vi "Main.vi"() -> ()   [LabVIEW 2018, in "Bookmark Manager.lvlib"]
uses:
  Bookmark Manager.lvlib
  Controls/State.ctl
  Controls/Bookmarks Groups.ctl
  Controls/Application Information.ctl
  Controls/VI Information.ctl
  Controls/VI Bookmark.ctl
  <vilib>/event_ctls.llb/eventvkey.ctl
panel:
  in  "Bookmarks Group":T1
  in  "Help":bool
  in  "Close":bool
  in  "Bookmarks":string(tree)
  in  "Scope":u16(ring) items=["Main Application Instance", "Eulogy", "Default Bookmark Manager with image"]
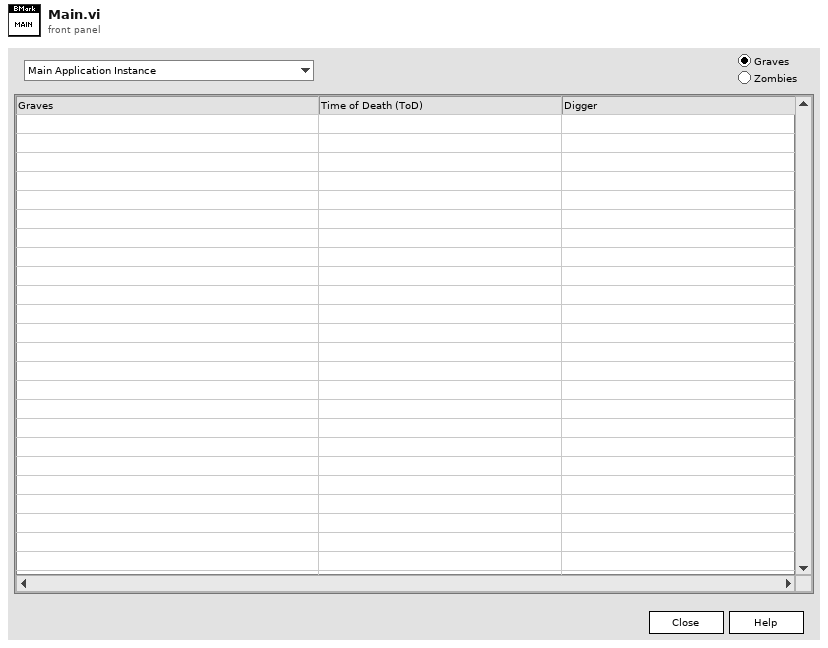
[diagram p1: front panel]
types:
  T1 = typedef "Bookmark Manager.lvlib/Bookmarks Groups.ctl" = enum32{"Graves", "Zombies"}
  T2 = typedef "Bookmark Manager.lvlib/State.ctl" = cluster{"Bookmarks":T3[], "Bookmarks Filter":T1, "Bookmarks Group":refnum<vi>, "Bookmarks View":refnum<vi>, "Front Panel":refnum<vi>, "Scopes":refnum<vi>}
  T3 = typedef "Bookmark Manager.lvlib/VI Bookmark.ctl" = cluster{"Bookmark Info":cluster{"Bookmark ID":u32, "Bookmark Tag":string, "Label Text":string}, "VI Info":T4}
  T4 = typedef "Bookmark Manager.lvlib/VI Information.ctl" = cluster{"App Info":T5, "Name":string, "Path":path}
  T5 = typedef "Bookmark Manager.lvlib/Application Information.ctl" = cluster{"Project":string, "Target":string}
  T6 = enum32{"Invalid", "Standard", "Closed", "Hidden", "Minimized", "Maximized"}
  T7 = typedef "eventvkey.ctl" = enum16{"ASCII", "Enter", "Return", "Shift", "Ctrl", "Alt", "Cmd", "Opt", "Caps", "NumLock", "Clear", "Break", "Up", "Down", "Left", "Right", "Insert", "Delete", "Home", "End", "PageUp", "PageDown", "Escape", "Help", "Pause", "ScrollLock", "F1", "F2", "F3", "F4", "F5", "F6", "F7", "F8", "F9", "F10", "F11", "F12", "F13", "F14", "F15", "F16", "F17", "F18", "F19", "F20", "F21", "F22", "F23", "F24", "Play", "VolumeUp", "VolumeDown", "Mute", "Two Byte Char"}
  T8 = typedef "LVPoint32TypeDef.ctl" = cluster{"Horizontal":i32, "Vertical":i32}
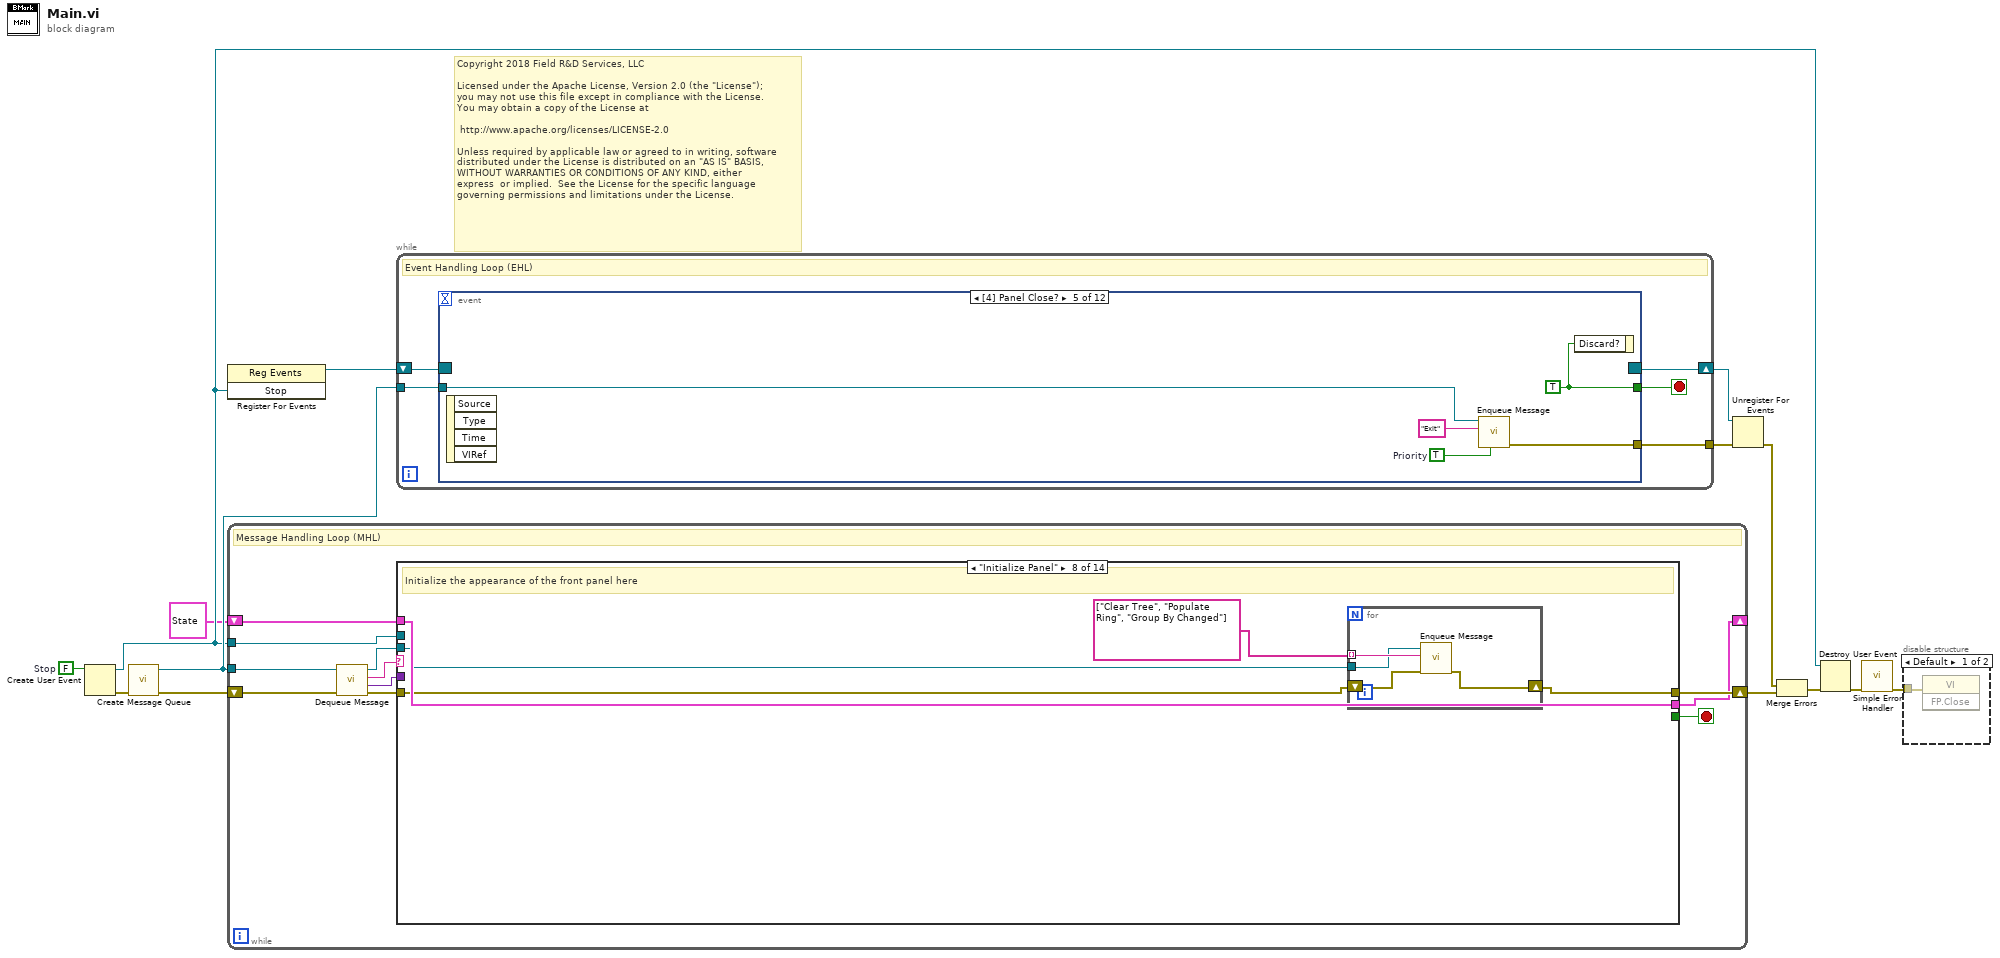
[diagram p0: block diagram]
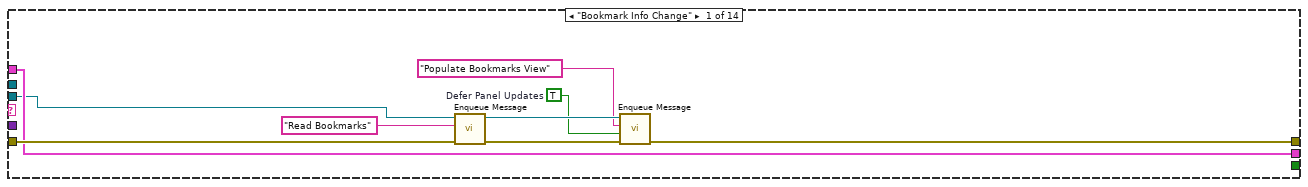
[diagram p3: hidden frame]
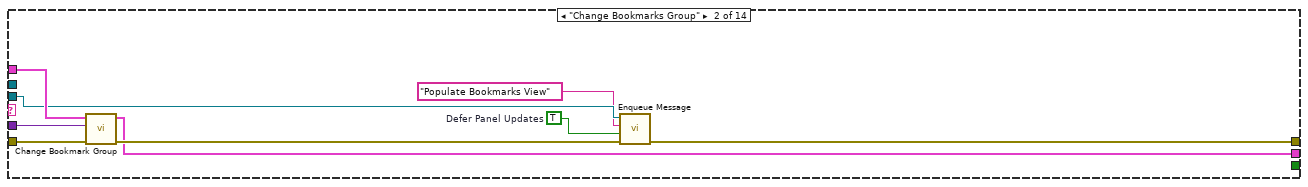
[diagram p4: hidden frame]
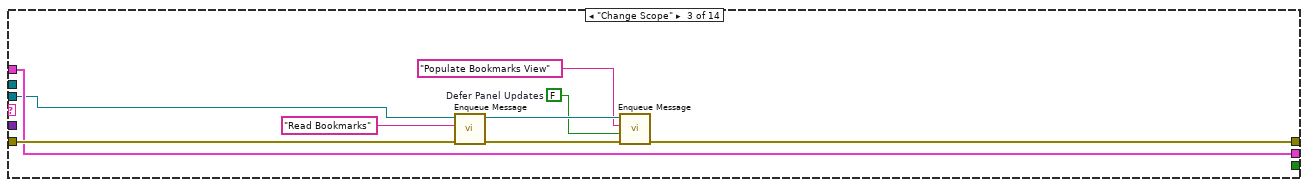
[diagram p5: hidden frame]
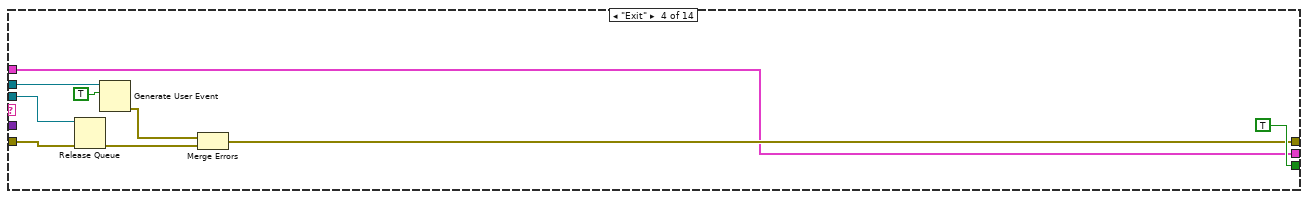
[diagram p6: hidden frame]
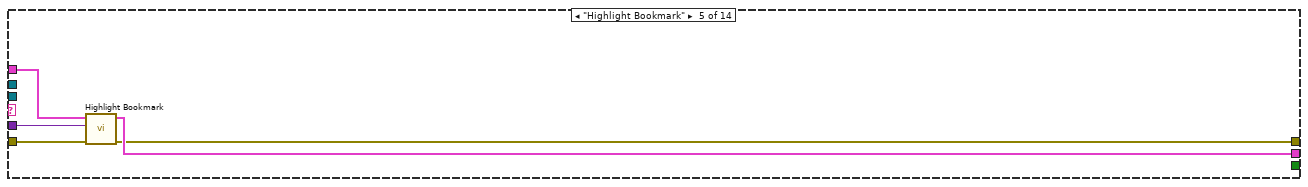
[diagram p7: hidden frame]
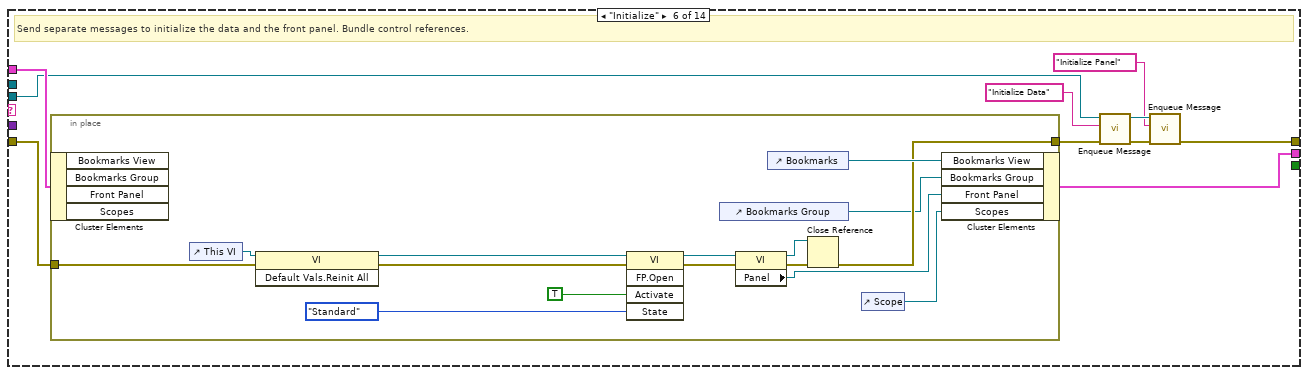
[diagram p8: hidden frame]
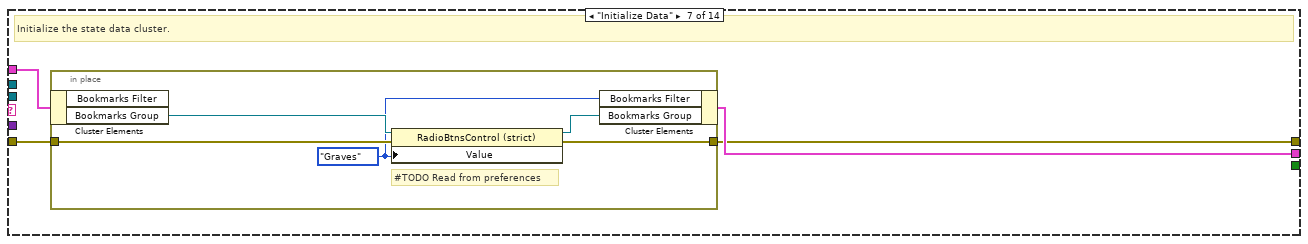
[diagram p9: hidden frame]
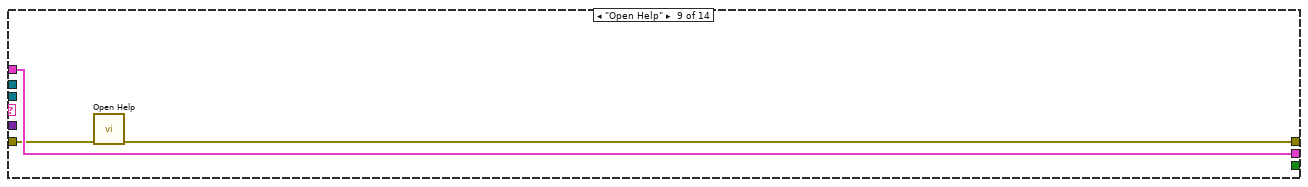
[diagram p10: hidden frame]
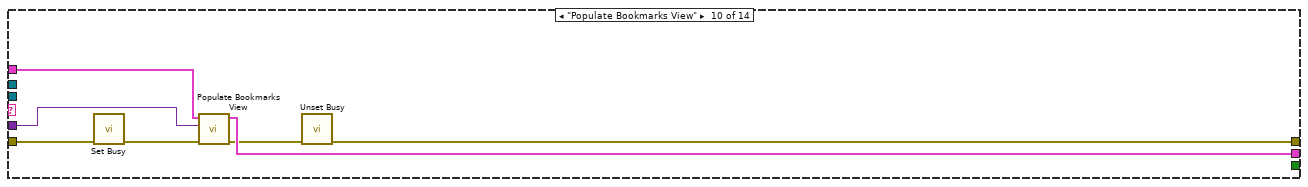
[diagram p11: hidden frame]
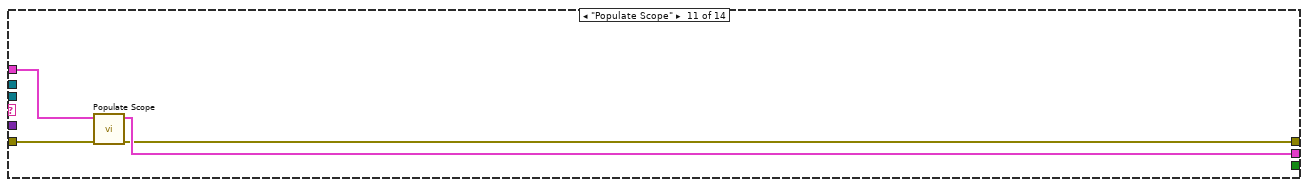
[diagram p12: hidden frame]
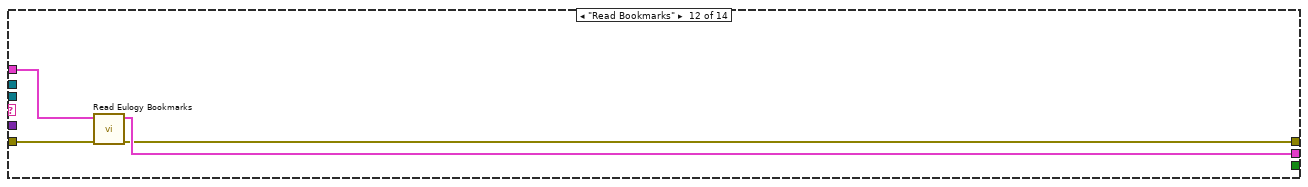
[diagram p13: hidden frame]
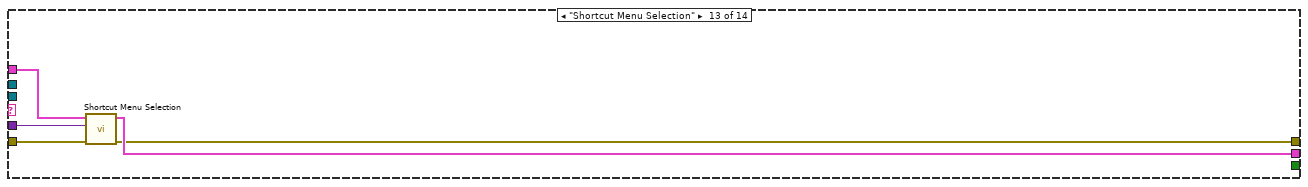
[diagram p14: hidden frame]
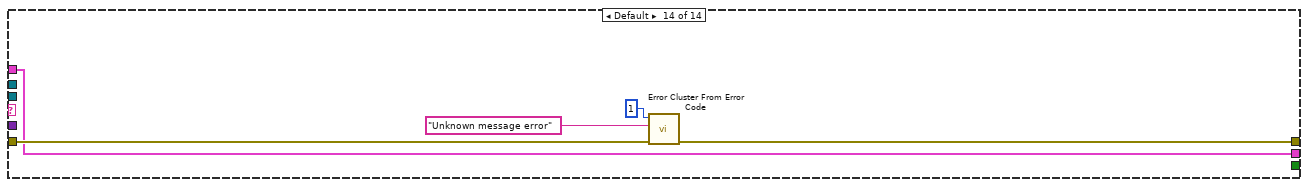
[diagram p15: hidden frame]
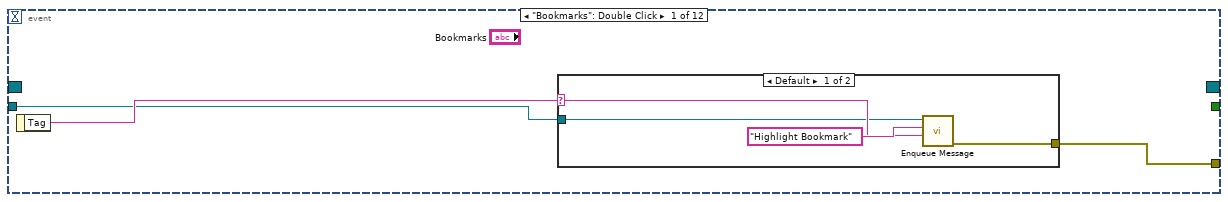
[diagram p16: hidden frame]
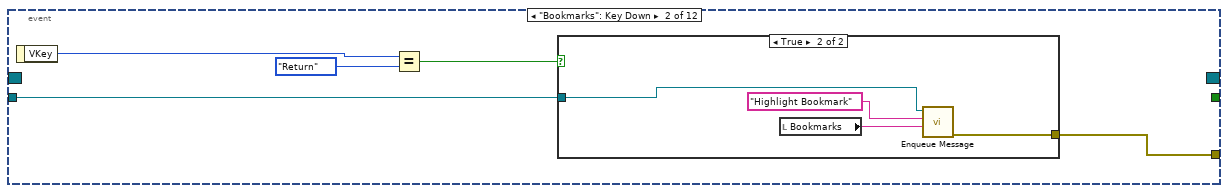
[diagram p18: hidden frame]
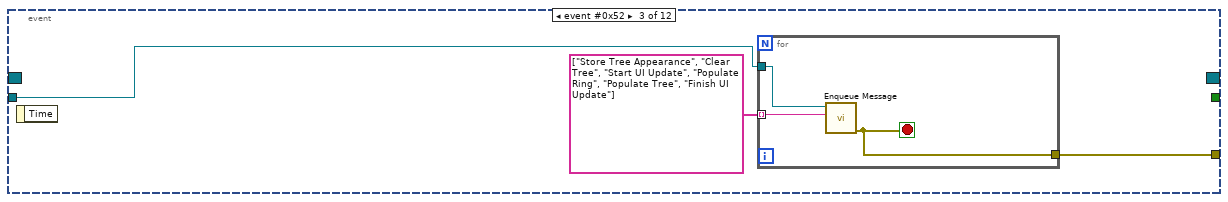
[diagram p20: hidden frame]
diagram:
  w12 = FALSE  # Stop
  # "Copyright 2018 Field R&D Services, LLC\n\nLicensed under the Apache License, Version 2.0 (the \"License\");\nyou may not use this file except in compliance with the License.\nYou may obtain a copy of the License at\n\n\thttp://www.apache.org/licenses/LICENSE-2.0\n\nUnless required by applicable law or agreed to in writing, software\ndistributed under the License is distributed on an \"AS IS\" BASIS,\nWITHOUT WARRANTIES OR CONDITIONS OF ANY KIND, either \nexpress  or implied.  See the License for the specific language \ngoverning permissions and limitations under the License."
  n1 = Create User Event(user event datatype=w12) -> (user event=w5:refnum<user-event>, error out=w11:errorcluster)  [unwired: 1 in]
  n2 = call "Create Message Queue.vi"("Error In"=w11) -> ("Error Out"=w9:errorcluster, "Message Queue"=w10:refnum<queue>)  [unwired: 9 in]
  n3 = register-events(w5) -> (reference out=w14:refnum<event-registration>)  [unwired: 2 in, 1 out]
  n4 = while {
    tunnel: w10 -> [w25]
    shift-right: [w23] -> w7
    shift-left: w9 -> [w22]
    tunnel: w5 -> [w19]
    shift-right: [w16] -> _
    shift-left: T2 {"Bookmarks"=[], "Bookmarks Filter"=enum."Graves", "Bookmarks Group"=refnum, "Bookmarks View"=refnum, "Front Panel"=refnum, "Scopes"=refnum} ("State") -> [w17]
    stop <- w20 stop-if-true
    # "Message Handling Loop (MHL)"
    n5 = call "Dequeue Message.vi"("Error In"=w22, "Message Queue In"=w25) -> ("Error Out"=w21:errorcluster, "Data"=w15:variant, "Command"=w24:string, "Message Queue Out"=w18:refnum<queue>)  [unwired: 6 in]
    n6 = case shown="\"Initialize Panel\"" w24 {
      tunnel: [w28 w38 w47 w59 w63 w68 w92 w101 w110 w114 w120 w124 w129 w133] -> w23
      tunnel: w21 -> [w34 w43 w52 w61 w66 w73 w93 w102 w111 w117 w121 w125 w132 w135]
      tunnel: [_ _ _ TRUE _ _ _ _ _ _ _ _ _ _] -> w20
      tunnel: w19 -> [_ _ _ w58 _ _ _ _ _ _ _ _ _ _]
      tunnel: w18 -> [w32 w37 w50 w54 _ w74 _ w103 _ _ _ _ _ _]
      tunnel: w17 -> [w33 w40 w51 w53 w62 w76 w95 w105 w112 w119 w123 w127 w131 w134]
      tunnel: [w33 w39 w51 w53 w64 w75 w94 w105 w112 w118 w122 w126 w130 w134] -> w16
      tunnel: w15 -> [_ w41 _ _ w65 _ _ _ _ w113 _ _ w128 _]
      frame "Bookmark Info Change" {
        w26 = TRUE  # Defer Panel Updates
        n7 = call "Enqueue Message.vi"("Error In"=w34, "Command"="Read Bookmarks", "Message Queue In"=w32) -> ("Error Out"=w30:errorcluster, "Message Queue Out"=w29:refnum<queue>)  [unwired: 7 in]
        n8 = call "Enqueue Message.vi"("Error In"=w30, "Data"=w26, "Command"="Populate Bookmarks View", "Message Queue In"=w29) -> ("Error Out"=w28:errorcluster)  [unwired: 6 in, 1 out]
      }
      frame "Change Bookmarks Group" {
        w35 = TRUE  # Defer Panel Updates
        n9 = call "Change Bookmark Group.vi"("Error In"=w43, "Data"=w41, "State In"=w40) -> ("Error Out"=w42:errorcluster, "State Out"=w39:T2)  [unwired: 7 in]
        n10 = call "Enqueue Message.vi"("Error In"=w42, "Data"=w35, "Command"="Populate Bookmarks View", "Message Queue In"=w37) -> ("Error Out"=w38:errorcluster)  [unwired: 6 in, 1 out]
      }
      frame "Change Scope" {
        w44 = FALSE  # Defer Panel Updates
        n11 = call "Enqueue Message.vi"("Error In"=w52, "Command"="Read Bookmarks", "Message Queue In"=w50) -> ("Error Out"=w48:errorcluster, "Message Queue Out"=w49:refnum<queue>)  [unwired: 7 in]
        n12 = call "Enqueue Message.vi"("Error In"=w48, "Data"=w44, "Command"="Populate Bookmarks View", "Message Queue In"=w49) -> ("Error Out"=w47:errorcluster)  [unwired: 6 in, 1 out]
      }
      frame "Exit" {
        n13 = Release Queue(queue=w54, error in (no error)=w61) -> (error out=w55:errorcluster)  [unwired: 1 in, 2 out]
        n14 = Generate User Event(user event=w58, event data cluster=TRUE ("event data")) -> (error out=w56:errorcluster)  [unwired: 2 in, 1 out]
        n15 = Merge Errors(w56, w55) -> (w59:errorcluster)
      }
      frame "Highlight Bookmark" {
        n16 = call "Highlight Bookmark.vi"("Error In"=w66, "Data"=w65, "State In"=w62) -> ("Error Out"=w63:errorcluster, "State Out"=w64:T2)  [unwired: 7 in]
      }
      frame "Initialize" {
        # "Send separate messages to initialize the data and the front panel. Bundle control references."
        n17 = in-place {
          in-place-border: w73 -> [w88]
          in-place-border: [w84] -> w72
          n18 = in-place-cluster #1(w76) -> ()  [unwired: 4 out]
          n19 = control-ref of="This VI"() -> (w85:refnum<vi>)
          n20 = invoke class="VI" method="Default Vals.Reinit All"(reference=w85, error in=w88) -> (reference out=w87:refnum<vi>, error out=w78:errorcluster)  [unwired: 1 in, 1 out]
          n21 = invoke class="VI" method="FP.Open"(reference=w87, error in=w78, "Activate"=TRUE ("Activate?"), "State"=T6."Standard") -> (reference out=w82:refnum<vi>, error out=w81:errorcluster)  [unwired: 1 in, 3 out]
          n22 = control-ref of="Bookmarks Group"() -> (w77:refnum<vi>)
          n23 = property class="VI"(reference=w82, error in=w81) -> (reference out=w83:refnum<vi>, error out=w86:errorcluster, "Panel"=w89:refnum<vi>)
          n24 = control-ref of="Bookmarks"() -> (w91:refnum<vi>)
          n25 = Close Reference(reference=w83, error in (no error)=w86) -> (error out=w84:errorcluster)
          n26 = control-ref of="Scope"() -> (w90:refnum<vi>)
          n27 = in-place-cluster #1("Bookmarks View"=w91, "Bookmarks Group"=w77, "Front Panel"=w89, "Scopes"=w90) -> (w75:T2)
        }
        n28 = call "Enqueue Message.vi"("Error In"=w72, "Command"="Initialize Data", "Message Queue In"=w74) -> ("Error Out"=w69:errorcluster, "Message Queue Out"=w71:refnum<queue>)  [unwired: 7 in]
        n29 = call "Enqueue Message.vi"("Error In"=w69, "Command"="Initialize Panel", "Message Queue In"=w71) -> ("Error Out"=w68:errorcluster)  [unwired: 7 in, 1 out]
      }
      frame "Initialize Data" {
        # "Initialize the state data cluster."
        n30 = in-place {
          in-place-border: w93 -> [w98]
          in-place-border: [w97] -> w92
          w96 = Bookmarks_Groups."Graves" ("Bookmarks Filter")
          # "#TODO Read from preferences"
          n31 = in-place-cluster #2(w95) -> ("Bookmarks Group"=w100:refnum<vi>)  [unwired: 1 out]
          n32 = property class="RadioBtnsControl (strict)"(reference=w100, error in=w98, "Value"=w96) -> (reference out=w99:refnum<vi>, error out=w97:errorcluster)
          n33 = in-place-cluster #2("Bookmarks Filter"=w96, "Bookmarks Group"=w99) -> (w94:T2)
        }
      }
      frame "Initialize Panel" {
        # "Initialize the appearance of the front panel here"
        n34 = for {
          tunnel: string[] ["Clear Tree", "Populate Ring", "Group By Changed"] -> [w109] mode=indexing
          tunnel: w103 -> [w108]
          shift-right: [w106] -> w101
          shift-left: w102 -> [w107]
          n35 = call "Enqueue Message.vi"("Error In"=w107, "Command"=w109, "Message Queue In"=w108) -> ("Error Out"=w106:errorcluster)  [unwired: 7 in, 1 out]
        }
      }
      frame "Open Help" {
        n36 = call "Open Help.vi"("Error In"=w111) -> ("Error Out"=w110:errorcluster)  [unwired: 10 in]
      }
      frame "Populate Bookmarks View" {
        n37 = call <vilib>:"Set Busy.vi"("error in (no error)"=w117) -> ("error out"=w115:errorcluster)  [unwired: 9 in, 1 out]
        n38 = call "Populate Bookmarks View.vi"("Error In"=w115, "Data"=w113, "State In"=w119) -> ("Error Out"=w116:errorcluster, "State Out"=w118:T2)  [unwired: 7 in]
        n39 = call <vilib>:"Unset Busy.vi"("error in (no error)"=w116) -> ("error out"=w114:errorcluster)  [unwired: 10 in]
      }
      frame "Populate Scope" {
        n40 = call "Populate Scope.vi"("Error In"=w121, "State In"=w123) -> ("Error Out"=w120:errorcluster, "State Out"=w122:T2)  [unwired: 8 in]
      }
      frame "Read Bookmarks" {
        n41 = call "Read Eulogy Bookmarks.vi"("Error In"=w125, "State In"=w127) -> ("Error Out"=w124:errorcluster, "State Out"=w126:T2)  [unwired: 8 in]
      }
      frame "Shortcut Menu Selection" {
        n42 = call "Shortcut Menu Selection.vi"("Error In"=w132, "Data"=w128, "State In"=w131) -> ("Error Out"=w129:errorcluster, "State Out"=w130:T2)  [unwired: 7 in]
      }
      frame Default {
        n43 = call <vilib>:"Error Cluster From Error Code.vi"("error in (no error)"=w135, "error message (\"\")"="Unknown message error" ("error message (\"\")"), "error code (0)"=1) -> ("error out"=w133:errorcluster)  [unwired: 6 in]
      }
    }
  }
  n44 = while {
    shift-right: [w141] -> w13
    shift-left: w14 -> [w142]
    tunnel: w10 -> [w140]
    tunnel: [w138] -> w1
    stop <- w139 stop-if-true
    # "Event Handling Loop (EHL)"
    n45 = event shown="[4] Panel Close?" {
      selector: w142 -> [_ _ _ _ _ _ _ _ _ _ _ _]
      dyn-events: [_ _ _ _ _ _ _ _ _ _ _ _] -> w141
      timeout: _ -> [_ _ _ _ _ _ _ _ _ _ _ _]
      tunnel: [_ _ _ _ w176 TRUE _ _ _ FALSE FALSE TRUE] -> w139
      tunnel: w140 -> [w144 w151 w161 w167 w173 w179 w183 w188 _ w197 w203 _]
      tunnel: [w143 w150 w159 w165 w172 w177 w182 w186 w189 w194 w199 _] -> w138
      event "Bookmarks": Double Click {
        n46 = event-data() -> ("Tag"=w145:string)  [unwired: 1 in]
        n47 = case shown="Default" w145 {
          selector: w145 -> [w147 _]
          tunnel: [w149 _] -> w143
          tunnel: w144 -> [w146 _]
          frame Default {
            n48 = call "Enqueue Message.vi"("Data"=w147, "Command"="Highlight Bookmark", "Message Queue In"=w146) -> ("Error Out"=w149:errorcluster)  [unwired: 7 in, 1 out]
          }
          frame "" {
          }
        }
      }
      event "Bookmarks": Key Down {
        n49 = event-data() -> ("VKey"=w154:T7)  [unwired: 1 in]
        n50 = Equal?(x=w154, y=eventvkey."Return") -> (x = y?=w152:bool)
        n51 = case shown="True" w152 {
          tunnel: w151 -> [_ w158]
          tunnel: [_ w155] -> w150
          frame False {
          }
          frame True {
            n52 = local read "Bookmarks"() -> (w156:string)
            n53 = call "Enqueue Message.vi"("Data"=w156, "Command"="Highlight Bookmark" ("Message"), "Message Queue In"=w158) -> ("Error Out"=w155:errorcluster)  [unwired: 7 in, 1 out]
          }
        }
      }
      event event #0x52 {
        n54 = event-data() -> ()  [unwired: 1 in, 1 out]
        n55 = for {
          tunnel: [w162] -> w159
          tunnel: w161 -> [w164]
          tunnel: string[] ["Store Tree Appearance", "Clear Tree", "Start UI Update", "Populate Ring", "Populate Tree", "Finish UI Update"] -> [w163] mode=indexing
          stop <- w162 stop-if-true
          n56 = call "Enqueue Message.vi"("Command"=w163, "Message Queue In"=w164) -> ("Error Out"=w162:errorcluster)  [unwired: 8 in, 1 out]
        }
      }
      event "Bookmarks": Shortcut Menu Selection (User) {
        n57 = event-data() -> ("ItemTag"=w166:string)  [unwired: 1 in]
        n58 = case shown="Default" w166 {
          selector: w166 -> [_ w168]
          tunnel: w167 -> [_ w171]
          tunnel: [_ w170] -> w165
          frame "" {
          }
          frame Default {
            n59 = call "Enqueue Message.vi"("Data"=w168, "Command"="Shortcut Menu Selection", "Message Queue In"=w171) -> ("Error Out"=w170:errorcluster)  [unwired: 7 in, 1 out]
          }
        }
      }
      event Panel Close? {
        w174 = TRUE  # Priority
        w176 = TRUE
        n60 = event-data() -> ()  [unwired: 1 in, 4 out]
        n61 = call "Enqueue Message.vi"("Priority"=w174, "Command"="Exit", "Message Queue In"=w173) -> ("Error Out"=w172:errorcluster)  [unwired: 7 in, 1 out]
        n62 = event-data("Discard?"=w176) -> ()  [unwired: 1 in, 1 out]
      }
      event Application Instance Close {
        w180 = TRUE  # Priority
        # "#TODO Add saving preferences"
        n63 = event-data() -> ()  [unwired: 1 in, 1 out]
        n64 = call "Enqueue Message.vi"("Priority"=w180, "Command"="Exit", "Message Queue In"=w179) -> ("Error Out"=w177:errorcluster)  [unwired: 7 in, 1 out]
      }
      event "Close": Value Change {
        w184 = TRUE  # Priority
        n65 = event-data() -> ()  [unwired: 1 in, 1 out]
        n66 = call "Enqueue Message.vi"("Priority"=w184, "Command"="Exit", "Message Queue In"=w183) -> ("Error Out"=w182:errorcluster)  [unwired: 7 in, 1 out]
      }
      event "Help": Value Change {
        n67 = event-data() -> ()  [unwired: 1 in, 1 out]
        n68 = call "Enqueue Message.vi"("Command"="Open Help", "Message Queue In"=w188) -> ("Error Out"=w186:errorcluster)  [unwired: 8 in, 1 out]
      }
      event "Bookmarks": Shortcut Menu Activation? {
        # "Dynamic menu generation must be handled within the EHL (producer) and this case specifically instead of the MHL (consumer) because the MenuRef's lifetime is only within this Event case. In other words, as soon as this Event case is over, the MenuRef becomes invalid. An error occurs if the menu is generated outside of this event case."
        n69 = event-data() -> ("MenuRef"=w192:refnum<k9>, "Coords"=w191:T8)  [unwired: 1 in]
        n70 = control-ref of="Bookmarks"() -> (w190:refnum<vi>)
        n71 = call "Bookmarks View Shortcut Menu Activation.vi"("Coords"=w191, "MenuRef"=w192, "TreeControl In"=w190) -> ("Error Out"=w189:errorcluster)  [unwired: 7 in, 1 out]
        n72 = event-data("Discard?"=FALSE) -> ()  [unwired: 1 in, 1 out]
      }
      event Value Change {
        n73 = event-data() -> ()  [unwired: 1 in, 1 out]
        n74 = call "Enqueue Message.vi"("Data"="Bookmarks Group", "Command"="Change Bookmarks Group", "Message Queue In"=w197) -> ("Error Out"=w194:errorcluster)  [unwired: 7 in, 1 out]
      }
      event "Scope": Value Change {
        n75 = event-data() -> ("NewVal"=w200:u16)  [unwired: 1 in]
        n76 = call "Enqueue Message.vi"("Data"=w200, "Command"="Change Scope", "Message Queue In"=w203) -> ("Error Out"=w199:errorcluster)  [unwired: 7 in, 1 out]
      }
      event User Event {
        n77 = event-data() -> ()  [unwired: 1 in, 1 out]
      }
    }
  }
  n78 = Unregister For Events(event registration refnum=w13, error in=w1) -> (error out=w8:errorcluster)
  n79 = Merge Errors(w8, w7) -> (w6:errorcluster)
  n80 = Destroy User Event(user event=w5, error in=w6) -> (error out=w4:errorcluster)
  n81 = call <vilib>:"Simple Error Handler.vi"("error in (no error)"=w4) -> ("error out"=w3:errorcluster)  [unwired: 4 in, 4 out]
  n82 = disable-structure shown="Default" {
    disable-tunnel: w3 -> [w205 _]
    frame condition #0 {
      n83 = invoke class="VI" method="FP.Close"(error in=w205) -> ()  [unwired: 2 in, 3 out]
    }
    frame condition #1 (active) {
    }
  }
